vi "processing subvi.vi"(9 "Operation":enum16{"sum", "sub", "multi", "div"}(ring), 10 "Input":dbl) -> (2 "Output":dbl)   [LabVIEW 2015]
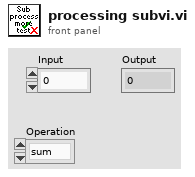
[diagram p1: front panel]
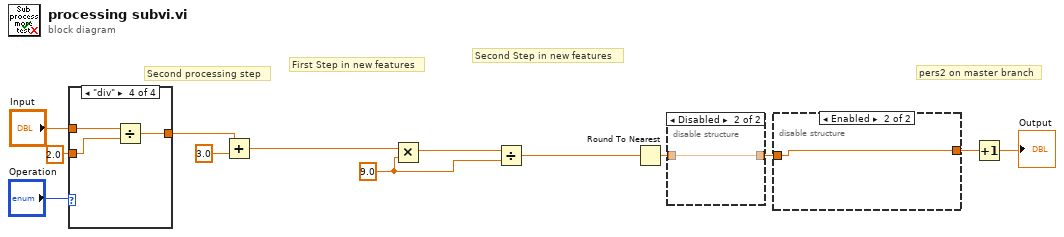
[diagram p0: block diagram]
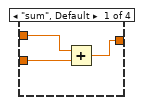
[diagram p2: hidden frame]
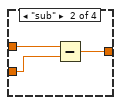
[diagram p3: hidden frame]
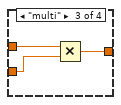
[diagram p4: hidden frame]
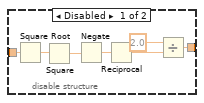
[diagram p5: hidden frame]
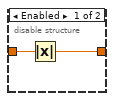
[diagram p6: hidden frame]
diagram:
  w8 = 9.0 ("y")
  # "pers2 on master branch"
  # "Second Step in new features"
  # "First Step in new features"
  # "Second processing step"
  n1 = case shown="\"div\"" "Operation" {
    tunnel: "Input" -> [w15 w19 w22 w25]
    tunnel: [w16 w18 w21 w24] -> w11
    tunnel: 2.0 ("y") -> [w14 w17 w20 w23]
    frame "sum", Default {
      n2 = Add(x=w15, y=w14) -> (x+y=w16:dbl)
    }
    frame "sub" {
      n3 = Subtract(x=w19, y=w17) -> (x-y=w18:dbl)
    }
    frame "multi" {
      n4 = Multiply(x=w22, y=w20) -> (x*y=w21:dbl)
    }
    frame "div" {
      n5 = Divide(x=w25, y=w23) -> (x/y=w24:dbl)
    }
  }
  n6 = Add(x=w11, y=3.0) -> (x+y=w10:dbl)
  n7 = Multiply(x=w10, y=w8) -> (x*y=w9:dbl)
  n8 = Divide(x=w9, y=w8) -> (x/y=w1:dbl)
  n9 = Round To Nearest(number=w1) -> (nearest integer value=w7:dbl)
  n10 = disable-structure shown="Disabled" {
    disable-tunnel: [w27 w28] -> w5
    disable-tunnel: w7 -> [w26 w28]
    frame Enabled {
      n11 = Absolute Value(x=w26) -> (abs(x)=w27:dbl)
    }
    frame Disabled {
    }
  }
  n12 = disable-structure shown="Enabled" {
    disable-tunnel: w5 -> [w35 w36]
    disable-tunnel: [w30 w36] -> w6
    frame Disabled {
      n13 = Square Root(x=w35) -> (sqrt(x)=w34:dbl)
      n14 = Square(x=w34) -> (x^2=w33:dbl)
      n15 = Negate(x=w33) -> (-x=w32:dbl)
      n16 = Reciprocal(x=w32) -> (1/x=w31:dbl)
      n17 = Divide(x=2.0, y=w31) -> (x/y=w30:dbl)
    }
    frame Enabled {
    }
  }
  n18 = Increment(x=w6) -> (x+1=→"Output":dbl)
